vi "Random (0 - 1) with Seed.vi"(9 "v_seeds_in":dbl[](array[numeric]), 10 "Tag.lvclass":refnum<class "Tag.lvclass">, 11 "h_seeds_in":dbl[](array[numeric])) -> (0 "seed_v_out":dbl[](array[numeric]), 1 "v_element":dbl, 2 "h_element":dbl, 3 "seed_h_out":dbl[](array[numeric]))   [LabVIEW 2014]
uses:
  Tag.lvclass
  <vilib>/gmath/statdist.llb/Uniform Random.vi
  <vilib>/gmath/NI_Gmath.lvlib
panel:
  # "TODO: h_element en seed_h_verandert niet"
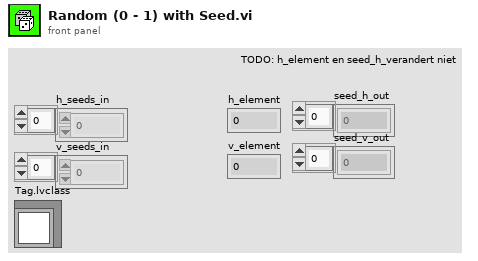
[diagram p1: front panel]
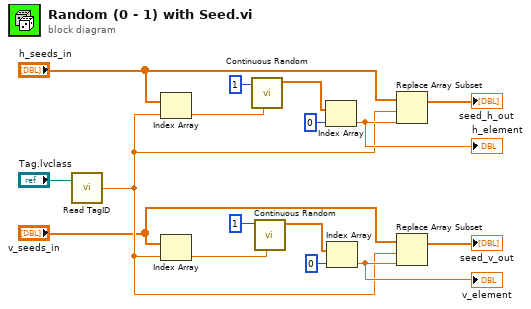
[diagram p0: block diagram]
diagram:
  n1 = call-dynamic "Read TagID.vi"("Tag in"="Tag.lvclass") -> ("TagID"=w3:dbl)  [unwired: 1 in, 2 out]
  n2 = Index Array(array="h_seeds_in", index=w3) -> (element=w14:dbl)
  n3 = Index Array(array="v_seeds_in", index=w3) -> (element=w7:dbl)
  n4 = call-poly <vilib>:"Continuous Random.vi"("seed"=w14, "samples"=1) -> ("uniform random data"=w11:dbl[])  [unwired: 8 in, 1 out]
  n5 = call-poly <vilib>:"Continuous Random.vi"("seed"=w7, "samples"=1) -> ("uniform random data"=w10:dbl[])  [unwired: 8 in, 1 out]
  n6 = Index Array(array=w11, index=0) -> (element=w5:dbl)
  "h_element" <- w5
  n7 = Index Array(array=w10, index=0) -> (element=w6:dbl)
  "v_element" <- w6
  n8 = Replace Array Subset(array="h_seeds_in", new element=w5, index=w3) -> (→"seed_h_out":dbl[])
  n9 = Replace Array Subset(array="v_seeds_in", new element=w6, index=w3) -> (→"seed_v_out":dbl[])
